vi "Labo-3-fin-partie3.vi"() -> ()   [LabVIEW 2020]
uses:
  <instrlib>/Agilent 34401/Public/Data/Read (Single Point).vi
  <instrlib>/Agilent E363X Series/Agilent E363X Series.lvlib
  <instrlib>/Agilent 34401/Agilent 34401.lvlib
panel:
  out "XY Graph":cluster{"Y":dbl[], "Y":dbl[]}[](graph) caption="Graphe XY"
  in  "Plage tension":dbl(slide) scale=0.0..4.0
  out "Courant":dbl
  in  "Incrément tension":dbl
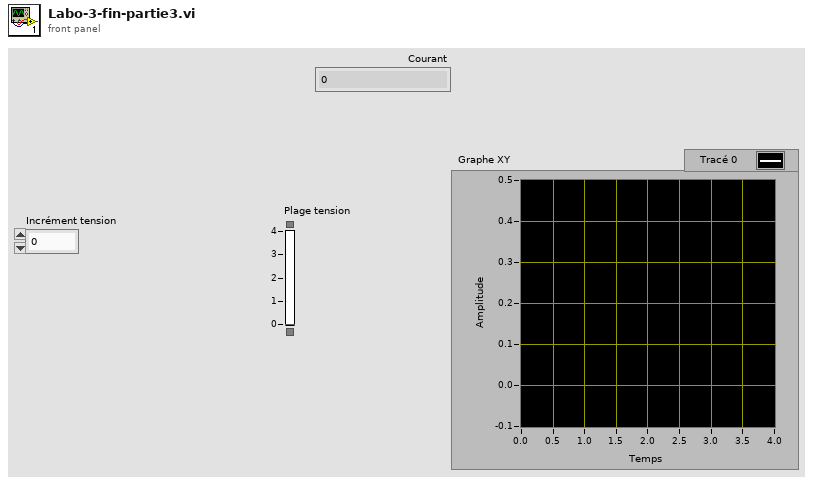
[diagram p1: front panel]
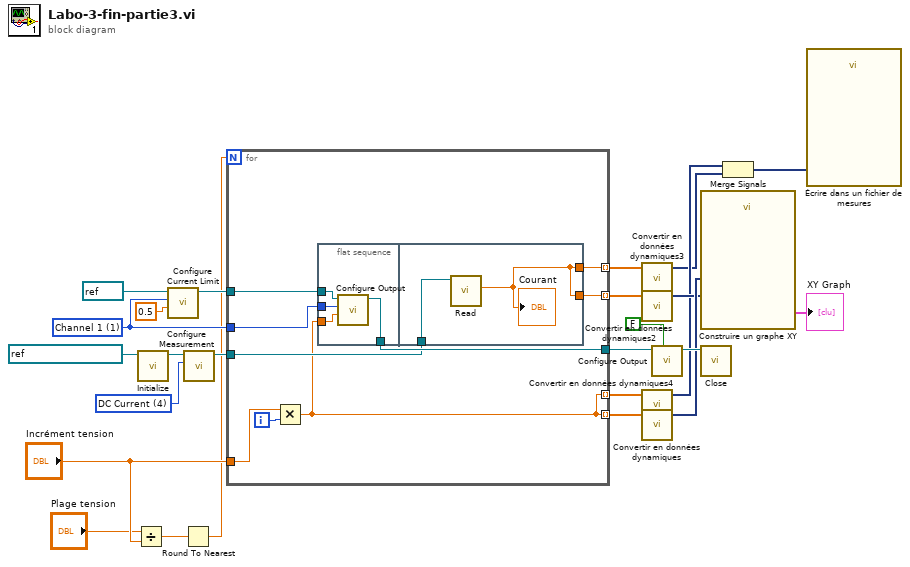
[diagram p0: block diagram]
diagram:
  w22 = u16 4 items=["DC Voltage", "AC Voltage", "2 - Wire Resistance", "4 - Wire Resistance", "DC Current", "AC Current", "Frequency", "Period", "Continuity", "Diode Checking", "VDC:VDC Ratio", "Temperature", "Capacitance"] ("Function (0: DC Voltage)")
  w19 = 1 items=["Channel 1"=1, "Channel 2"=2, "Channel 3"=3] ("Channel (1: Channel 1)")
  n1 = Divide(x="Plage tension", y="Incrément tension") -> (x/y=w13:dbl)
  n2 = call <instrlib>:"Initialize.vi"("VISA resource name"=refnum<visa-resource-name> "GPIB0::22::INSTR") -> ("VISA resource name out"=w23:refnum<visa-resource-name>)  [unwired: 9 in, 1 out]
  n3 = call <instrlib>:"Configure Current Limit.vi"("Current Limit (0.0 A)"=0.5, "Channel (1: Channel 1)"=w19, "VISA resource name"=refnum<visa-resource-name> "GPIB0::5::INSTR") -> ("VISA resource name out"=w18:refnum<visa-resource-name>)  [unwired: 7 in, 1 out]
  n4 = Round To Nearest(number=w13) -> (nearest integer value=w12:dbl)
  n5 = call <instrlib>:"Configure Measurement.vi"("Function (0: DC Voltage)"=w22, "VISA resource name"=w23) -> ("VISA resource name out"=w16:refnum<visa-resource-name>)  [unwired: 8 in, 1 out]
  n6 = for {
    N: w12 -> [_]
    tunnel: w19 -> [w34]
    tunnel: w18 -> [w33]
    tunnel: [w32] -> w17
    tunnel: w16 -> [w31]
    tunnel: "Incrément tension" -> [w30]
    tunnel: [w26] -> w10 mode=indexing
    tunnel: [w28] -> w8 mode=indexing
    tunnel: [w27] -> w6 mode=indexing
    tunnel: [w26] -> w5 mode=indexing
    i -> [w29]
    n7 = Multiply(x=w30, y=w29) -> (x*y=w26:dbl)
    n8 = flat-sequence {
      tunnel: w34 -> [w38]
      tunnel: w33 -> [w37]
      tunnel: [w36] -> w32
      tunnel: w26 -> [w35]
      tunnel: w31 -> [w40]
      tunnel: [w39] -> w28
      tunnel: [w39] -> w27
      frame #0 {
        n9 = call <instrlib>:"Configure Output.vi"("Voltage Level (0.0 V)"=w35, "Channel (1: Channel 1)"=w38, "VISA resource name"=w37) -> ("VISA resource name out"=w36:refnum<visa-resource-name>)  [unwired: 7 in, 1 out]
      }
      frame #1 {
        n10 = call-poly <instrlib>:"Read.vi"("VISA resource name"=w40) -> ("Measurement"=w39:dbl)  [unwired: 8 in, 2 out]
        "Courant" <- w39
      }
    }
  }
  n11 = call "Convertir en données dynamiques3"("Array"=w6) -> ("Dynamic Data Type"=w2:dynamicdata)  [unwired: 3 in]
  n12 = call "Convertir en données dynamiques2"("Array"=w8) -> ("Dynamic Data Type"=w7:dynamicdata)  [unwired: 3 in]
  n13 = call "Convertir en données dynamiques4"("Array"=w5) -> ("Dynamic Data Type"=w3:dynamicdata)  [unwired: 3 in]
  n14 = call "Convertir en données dynamiques"("Array"=w10) -> ("Dynamic Data Type"=w9:dynamicdata)  [unwired: 3 in]
  n15 = call <instrlib>:"Configure Output.vi"("Enable Output (T: Enable)"=FALSE, "VISA resource name"=w17) -> ("VISA resource name out"=w20:refnum<visa-resource-name>)  [unwired: 8 in, 1 out]
  n16 = call "Construire un graphe XY"("Y Input"=w7, "X Input"=w9) -> ("XY Graph"=→"XY Graph":cluster{"X":dbl[], "Y":dbl[]}[])  [unwired: 8 in, 1 out]
  n17 = call <instrlib>:"Close.vi"("VISA resource name"=w20) -> ()  [unwired: 10 in, 1 out]
  n18 = Merge Signals(w3, w2) -> (w4:dynamicdata)
  n19 = call "Écrire dans un fichier de mesures"("Signals"=w4) -> ()  [unwired: 16 in, 3 out]
